vi "Write_To_File.vi"(8 "error in":errorcluster, 10 "data":string, 11 "cookie":string) -> (0 "error out":errorcluster, 3 "path":path)   [LabVIEW 2015]
doc: "Writes events data to a file with name equal to the client sessions cookie"
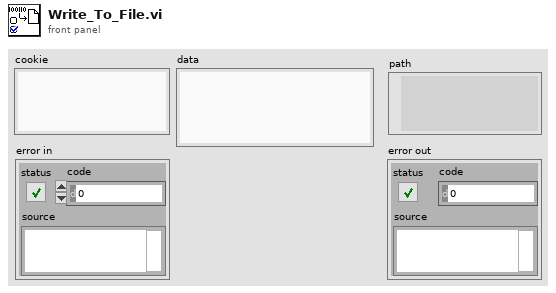
[diagram p1: front panel]
types:
  T1 = enum16{"open", "replace", "create", "open or create", "replace or create", "replace or create with confirmation"}
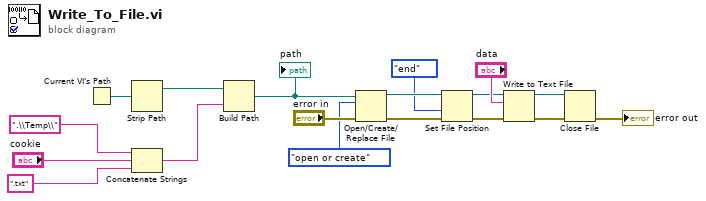
[diagram p0: block diagram]
diagram:
  n1 = Current VI's Path() -> (path=w9:path)
  n2 = Strip Path(path=w9) -> (stripped path=w8:path)  [unwired: 1 out]
  n3 = Concatenate Strings(".\\Temp\\", "cookie", ".txt" ("string")) -> (w7:string)
  n4 = Build Path(base path=w8, name or relative path=w7) -> (appended path=w6:path)
  "path" <- w6
  n5 = Open/Create/Replace File(file path (use dialog)=w6, error in="error in", operation (0:open)=T1."open or create") -> (refnum out=w5:refnum<file>, error out=w3:errorcluster)  [unwired: 3 in, 1 out]
  n6 = Set File Position(refnum=w5, from (0:start)=enum16{"start", "end", "current"}."end", error in=w3) -> (refnum out=w4:refnum<file>, error out=w2:errorcluster)  [unwired: 1 in]
  n7 = Write to Text File(file (use dialog)=w4, text="data", error in=w2) -> (refnum out=w17:refnum<file>, error out=w18:errorcluster)  [unwired: 1 in, 1 out]
  n8 = Close File(refnum=w17, error in=w18) -> (error out=→"error out":errorcluster)  [unwired: 1 out]
